vi "STMmyRIO-Server.vi"() -> ()   [LabVIEW 2015]
uses:
  <vilib>/NI/STM/SubVIs/MetaDataElement.ctl
  <vilib>/NI/STM/TCP/TCP Read Options.ctl
  <vilib>/NI/STM/TCP/Write Meta Data (TCP Ref).vi
  <vilib>/NI/STM/TCP/Get Connection Reference (TCP).vi
  <vilib>/NI/STM/TCP/Write Meta Data (TCP Clst).vi
  <vilib>/NI/STM/TCP/Read Message (TCP).vi
  <vilib>/NI/STM/TCP/Write Message (TCP).vi
  <vilib>/NI/STM/NI STM.lvlib
panel:
  out "手动取点y":i32
  out "手动取点x":i32
  out "是否手动取点":bool
  in  "?":bool
  in  "?":bool
  in  "?":bool
  out "触发":bool
  out "自动后退":bool
  out "自动前进":bool
  out "步进距离":u16
  in  "阈值等级":i32=4
  in  "Stop (F)":bool
  in  "关闭程序":bool
  out "error  out":errorcluster
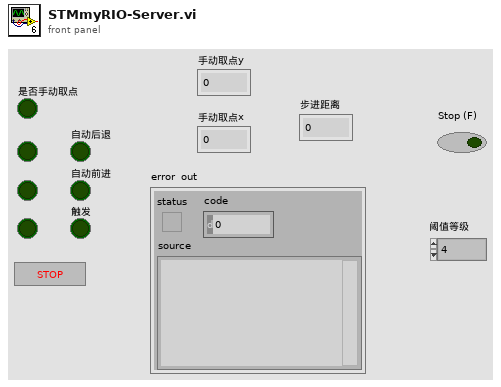
[diagram p1: front panel]
types:
  T1 = typedef "NI STM.lvlib/MetaDataElement.ctl" = string
  T2 = typedef "NI STM.lvlib/TCP Connection Info.ctl" = cluster{"connection ID":refnum<k5>, "meta data":T1[]}
  T3 = cluster{"图像数据":refnum<queue>, "队列输出":refnum<queue>}
  T4 = typedef "IMAQ Image.ctl" = refnum<image>
  T5 = cluster{"滤波":T4, "边缘检测":T4, "untitled":T4, "3D view":T4, "灰度图像":T4}
  T6 = cluster{"周长":dbl, "面积":dbl, "3D":u8[], "灰度图像":T4, "3D view":T4, "滤波":T4, "边缘检测":T4, "3D图像":T4, "质心坐标X":sgl, "质心坐标Y":sgl, "第一点y值，x=0":dbl, "第二点y值，x=639":dbl, "第一点x值，y=0":dbl, "第二点x值，y=479":dbl, "短轴半径um":dbl, "长轴半径um":dbl, "长轴长度":dbl, "短轴长度":dbl, "短轴原曲线":dbl[], "长轴拟合":dbl[], "纵轴拟合":dbl[], "横轴拟合":dbl[], "长轴原曲线":dbl[], "纵轴原曲线":dbl[], "横轴原曲线":dbl[], "短轴拟合":dbl[], "位置":dbl, "触发":bool, "初始化后退":bool, "初始化前进":bool}
  T7 = typedef "NI STM.lvlib/TCP Read Options.ctl" = cluster{"ignore timeout error":bool, "timeout ms (1000)":i32}
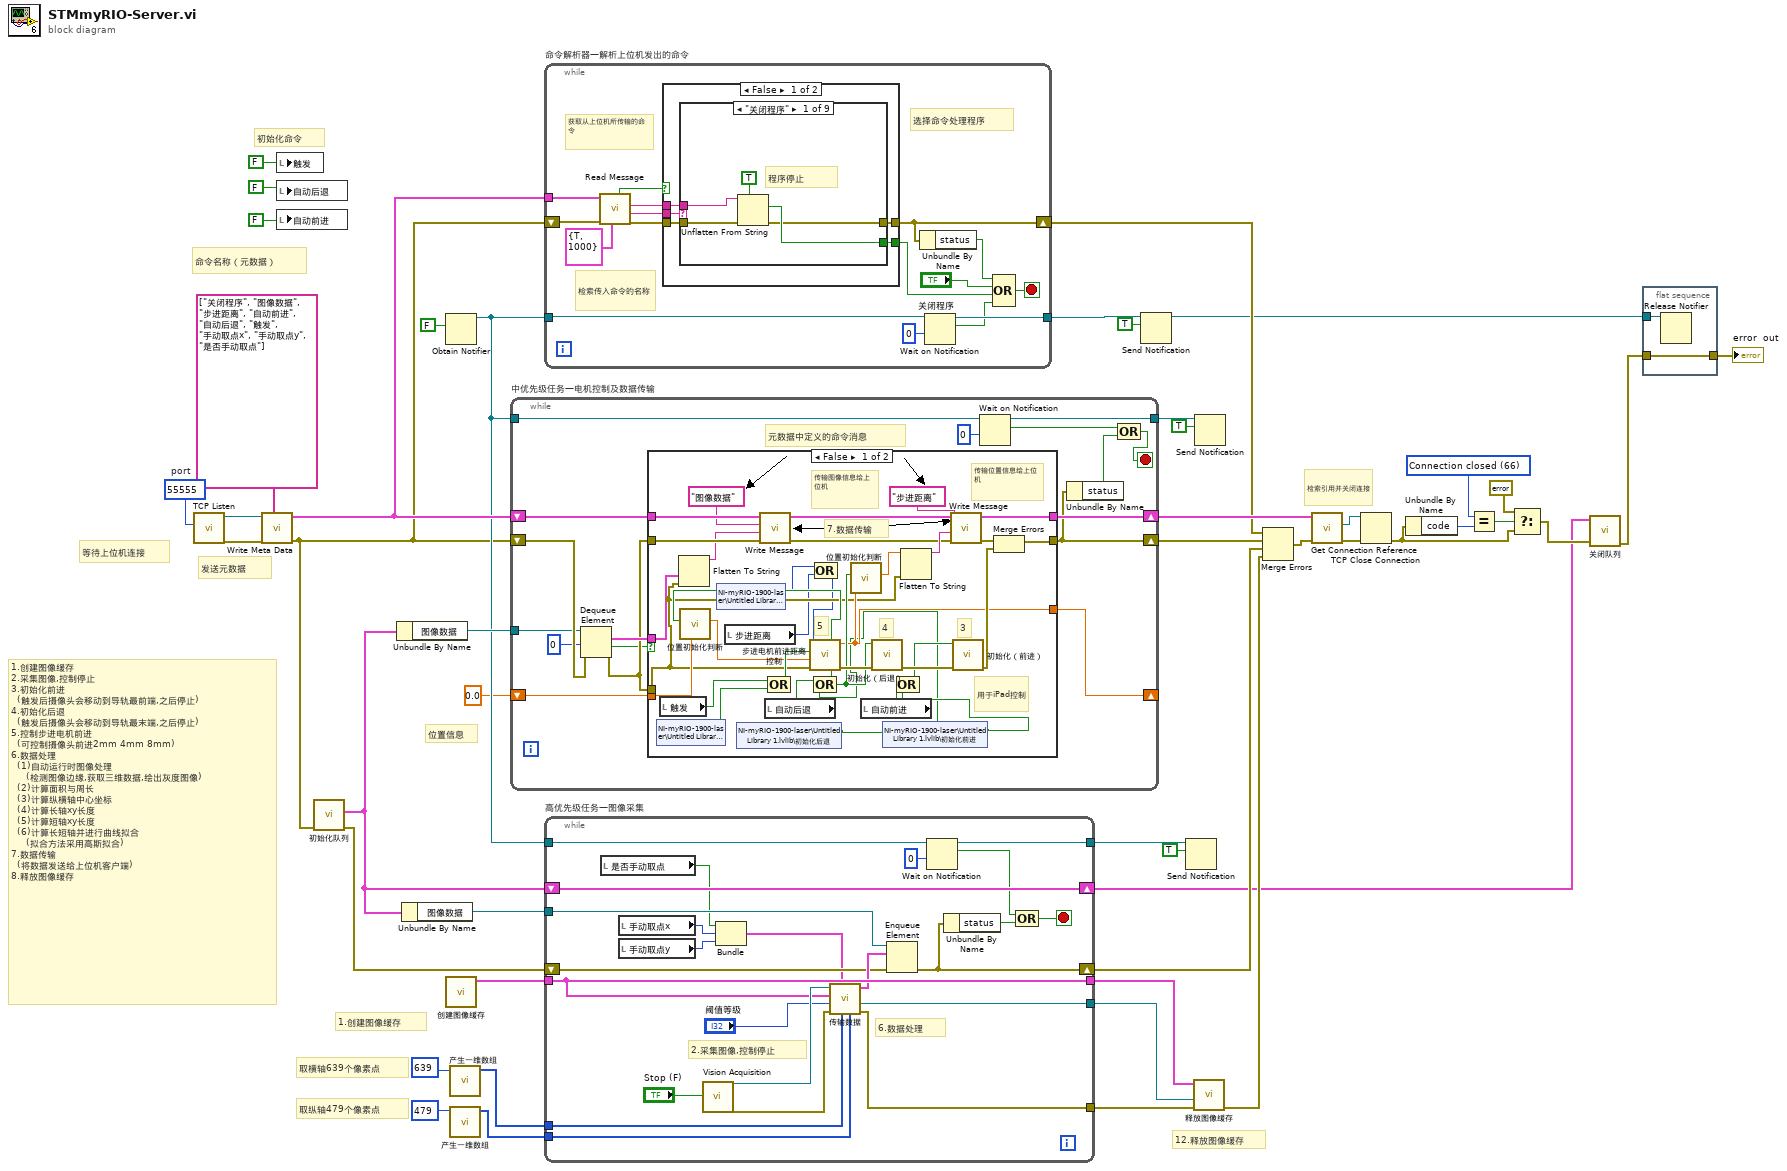
[diagram p0: block diagram]
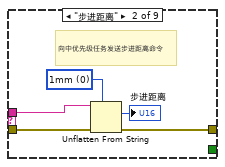
[diagram p3: hidden frame]
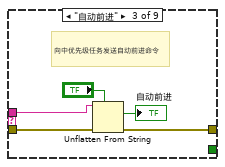
[diagram p4: hidden frame]
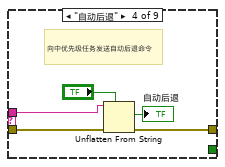
[diagram p5: hidden frame]
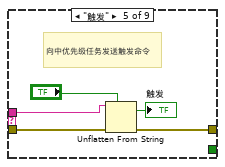
[diagram p6: hidden frame]
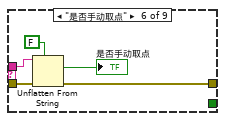
[diagram p7: hidden frame]
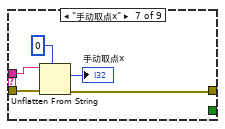
[diagram p8: hidden frame]
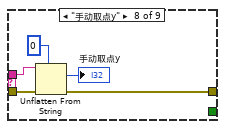
[diagram p9: hidden frame]
diagram:
  w22 = 66 items=["No Error", "Argument Error", "Memory Full", "Out of Zone", "End of File", "File Already Open", "Generic File IO Error", "File Not Found", "File Permission Error", "Disk Full", "Duplicate Path", "Too Many Files Open", "Not Enabled", "Resource File Not Found", "Cannot Add Resource", "Resource Not Found", "Image Not Found", "Image Memory Error", "Pen Does Not Exist", "Config Bad Type", "Config Token Not Found", "Config Parse Error", "Config Memory Error", "Bad External Code Format", "Bad External Code Offset", "External Code Not Present", "Null Window", "Destroy Window Mixup", "Null Menu", "Print Aborted", "Bad Print Record", "Print Driver Error", "Windows Error During Print", "Memory Error During Print", "Print Dialog Error", "Generic Print Error", "Invalid Device Refnum", "Device Not Found", "Device Parameter Error", "Device Unit Error", "Can't Open Device", "Device Call Aborted", "Generic Error", "Cancelled By User", "Object ID Too Low", "Object ID Too High", "Object Not In Heap", "Unknown Heap", "Bad DefProc ID", "DefProc Not In Table", "Message Out Of Range", "Null Method", "Unknown Message", "Manager Call Not Supported", "Bad address", "Connection In progress", "Connection timed out", "Connection is already in progress", "Network attribute not supported", "Network error", "Address in use", "System out of memory", "Connection aborted", "Connection refused", "Connection is not connected", "Connection is already connected", "Connection closed", "Initialize error (interapplication manager)", "Bad occurrence", "Wait on unbound occurrence handler", "Occurrence queue overflow", "Bad path", "Semaphore not signaled", "Unrecognized type (interapplication manager)"] ("1st Error to Convert")
  w48 = u16 55555  # port
  # "位置信息"
  # "初始化命令"
  # "等待上位机连接"
  # "发送元数据"
  # "检索引用并关闭连接"
  # "命令名称（元数据）"
  # "1.创建图像缓存"
  # "1.创建图像缓存\n2.采集图像,控制停止\n3.初始化前进\n  (触发后摄像头会移动到导轨最前端,之后停止)\n4.初始化后退\n  (触发后摄像头会移动到导轨最末端,之后停止)\n5.控制步进电机前进\n  (可控制摄像头前进2mm 4mm 8mm)\n6.数据处理\n  (1)自动运行时图像处理\n     (检测图像边缘,获取三维数据,绘出灰度图像)\n  (2)计算面积与周长\n  (3)计算纵横轴中心坐标\n  (4)计算长轴xy长度\n  (5)计算短轴xy长度\n  (6)计算长短轴并进行曲线拟合\n     (拟合方法采用高斯拟合) \n7.数据传输 \n  (将数据发送给上位机客户端) \n8.释放图像缓存"
  # "取纵轴479个像素点"
  # "取横轴639个像素点"
  # "12.释放图像缓存"
  n1 = call <vilib>:"TCP Listen.vi"("port"=w48) -> ("error out"=w46:errorcluster, "connection ID"=w47:refnum<k5>)  [unwired: 3 in, 6 out]
  n2 = call-poly "Write Meta Data.vi"("meta data"=T1[] ["关闭程序", "图像数据", "步进距离", "自动前进", "自动后退", "触发", "手动取点x", "手动取点y", "是否手动取点"] ("Meta data"), "error in"=w46, "connection ID"=w47) -> ("error out"=w19:errorcluster, "connection info out"=w45:T2)  [unwired: 2 in, 5 out]
  n3 = local write "触发"(FALSE) -> ()
  n4 = local write "自动后退"(FALSE) -> ()
  n5 = local write "自动前进"(FALSE) -> ()
  n6 = call "初始化队列.vi"("error in (no error)"=w19) -> ("error out"=w18:errorcluster, "输出簇"=w1:T3)  [unwired: 9 in]
  n7 = Unbundle By Name(w1) -> ("图像数据"=w44:refnum<queue>)
  n8 = Unbundle By Name(w1) -> ("图像数据"=w43:refnum<queue>)
  n9 = Obtain Notifier(notification data type=FALSE) -> (notifier out=w29:refnum<notifier>)  [unwired: 3 in, 2 out]
  n10 = call "创建图像缓存.vi"() -> ("簇"=w17:T5)  [unwired: 11 in]
  n11 = call "产生一维数组.vi"("Numeric"=639) -> ("Array"=w8:i32[])  [unwired: 10 in]
  n12 = call "产生一维数组.vi"("Numeric"=479) -> ("Array"=w7:i32[])  [unwired: 10 in]
  n13 = while "中优先级任务—电机控制及数据传输" {
    tunnel: w44 -> [w56]
    shift-right: [w58] -> w39
    shift-left: w19 -> [w62]
    shift-right: [w64] -> w42
    shift-left: w45 -> [w65]
    tunnel: w29 -> [w59]
    tunnel: [w57] -> w30
    shift-right: [w54] -> _
    shift-left: 0.0 ("x") -> [w55]
    stop <- w49 stop-if-true
    # "元数据中定义的命令消息"
    n14 = Dequeue Element(queue=w56, timeout in ms (-1)=0, error in (no error)=w62) -> (element=w63:T6, timed out?=w52:bool, error out=w53:errorcluster)  [unwired: 1 out]
    n15 = case shown="False" w52 {
      tunnel: w65 -> [w97 w100]
      tunnel: w53 -> [w96 w99]
      tunnel: [w89 w100] -> w64
      tunnel: [w84 w99] -> w58
      tunnel: w63 -> [w83 _]
      tunnel: w55 -> [w76 w98]
      tunnel: [w73 w98] -> w54
      tunnel: w53 -> [w71 _]
      frame False {
        # "传输图像信息给上位机"
        # "用于iPad控制"
        # "传输位置信息给上位机"
        # "7.数据传输"
        # "3"
        # "4"
        # "5"
        n16 = shared-variable "NI-myRIO-1900-laser\\Untitled Library 1.lvlib\\触发"() -> (w81:bool)  [unwired: 1 in, 1 out]
        n17 = local read "触发"() -> (w82:bool)
        n18 = Flatten To String(anything=w83, error in (no error)=w71) -> (data string=w94:string)  [unwired: 4 out]
        n19 = shared-variable "NI-myRIO-1900-laser\\Untitled Library 1.lvlib\\枚举"() -> (w66:i8)  [unwired: 1 in, 1 out]
        n20 = local read "步进距离"() -> (w68:u16)
        n21 = shared-variable "NI-myRIO-1900-laser\\Untitled Library 1.lvlib\\初始化后退"() -> (w69:bool)  [unwired: 1 in, 1 out]
        n22 = call-poly "Write Message.vi"("error in"=w96, "data"=w94, "name"="图像数据" ("Name"), "connection info in"=w97) -> ("error out"=w90:errorcluster, "connection info out"=w91:T2)  [unwired: 1 in, 5 out]
        n23 = local read "自动后退"() -> (w79:bool)
        n24 = Compound Arithmetic op=OR(w82, w81) -> (w80:bool)
        n25 = Compound Arithmetic op=OR(w79, w69) -> (w74:bool)
        n26 = call "位置初始化判断.vi"("位置初始化"=w76, "是否后退"=w74) -> ("位置判断"=w75:dbl)  [unwired: 9 in]
        n27 = Compound Arithmetic op=OR(w66, w68) -> (w67:u16)
        n28 = call "步进电机前进距离控制.vi"("error in"=w71, "初始化位置"=w75, "触发"=w80, "枚举"=w67) -> ("error out"=w88:errorcluster, "位置"=w73:dbl)  [unwired: 6 in]
        n29 = call "位置初始化判断.vi"("位置初始化"=w73, "是否后退"=w74) -> ("位置判断"=w72:dbl)  [unwired: 9 in]
        n30 = local read "自动前进"() -> (w78:bool)
        n31 = call "初始化（后退）.vi"("error in"=w88, "初始化"=w74) -> ("error out"=w87:errorcluster)  [unwired: 9 in]
        n32 = shared-variable "NI-myRIO-1900-laser\\Untitled Library 1.lvlib\\初始化前进"() -> (w70:bool)  [unwired: 1 in, 1 out]
        n33 = Compound Arithmetic op=OR(w78, w70) -> (w77:bool)
        n34 = Flatten To String(anything=w72, error in (no error)=w71) -> (data string=w93:string)  [unwired: 4 out]
        n35 = call-poly "Write Message.vi"("error in"=w90, "data"=w93, "name"="步进距离" ("Name"), "connection info in"=w91) -> ("error out"=w86:errorcluster, "connection info out"=w89:T2)  [unwired: 1 in, 5 out]
        n36 = call "初始化（前进）.vi"("error in"=w87, "初始化"=w77) -> ("error out"=w85:errorcluster)  [unwired: 9 in]
        n37 = Merge Errors(w86, w85) -> (w84:errorcluster)
      }
      frame True {
      }
    }
    n38 = Wait on Notification(notifier=w59, timeout in ms (-1)=0) -> (notifier out=w57:refnum<notifier>, notification=w51:bool)  [unwired: 2 in, 2 out]
    n39 = Unbundle By Name(w58) -> ("status"=w50:bool)
    n40 = Compound Arithmetic op=OR(w51, w50) -> (w49:bool)
  }
  n41 = while "命令解析器—解析上位机发出的命令" {
    tunnel: w45 -> [w116]
    shift-right: [w107] -> w37
    shift-left: w19 -> [w115]
    tunnel: w29 -> [w109]
    tunnel: [w103] -> w33
    stop <- w104 stop-if-true
    # "选择命令处理程序"
    # "检索传入命令的名称"
    # "获取从上位机所传输的命令"
    n42 = call-poly <vilib>:"Read Message.vi"("options"=T7 {"ignore timeout error"=TRUE, "timeout ms (1000)"=1000} ("Options"), "error in"=w115, "connection info in"=w116) -> ("error out"=w111:errorcluster, "name"=w114:T1, "data string"=w113:string, "timed out?"=w112:bool)  [unwired: 2 in, 3 out]
    n43 = case shown="False" w112 {
      tunnel: w114 -> [w117 _]
      tunnel: w113 -> [w121 _]
      tunnel: w111 -> [w120 w163]
      tunnel: [w119 w163] -> w107
      tunnel: [w118 _] -> w101
      frame False {
        n44 = case shown="\"关闭程序\"" w117 {
          tunnel: w121 -> [w125 w128 w135 w140 w145 w150 w154 w161 _]
          tunnel: w120 -> [w124 w131 w136 w141 w146 w149 w155 w160 w162]
          tunnel: [w122 w130 w134 w139 w144 w147 w153 w158 w162] -> w119
          tunnel: [w123 _ _ _ _ _ _ _ _] -> w118
          frame "关闭程序" {
            # "程序停止"
            n45 = Unflatten From String(type=TRUE, binary string=w125, error in (no error)=w124) -> (value=w123:bool, error out=w122:errorcluster)  [unwired: 1 in, 2 out]
          }
          frame "步进距离" {
            w129 = u16 0 items=["1mm", "2mm", "4mm", "8mm"] ("步进距离")
            # "向中优先级任务发送步进距离命令"
            n46 = Unflatten From String(type=w129, binary string=w128, error in (no error)=w131) -> (value=→"步进距离":u16, error out=w130:errorcluster)  [unwired: 1 in, 2 out]
          }
          frame "自动前进" {
            # "向中优先级任务发送自动前进命令"
            n47 = Unflatten From String(type="?", binary string=w135, error in (no error)=w136) -> (value=→"自动前进":bool, error out=w134:errorcluster)  [unwired: 1 in, 2 out]
          }
          frame "自动后退" {
            # "向中优先级任务发送自动后退命令"
            n48 = Unflatten From String(type="?", binary string=w140, error in (no error)=w141) -> (value=→"自动后退":bool, error out=w139:errorcluster)  [unwired: 1 in, 2 out]
          }
          frame "触发" {
            # "向中优先级任务发送触发命令"
            n49 = Unflatten From String(type="?", binary string=w145, error in (no error)=w146) -> (value=→"触发":bool, error out=w144:errorcluster)  [unwired: 1 in, 2 out]
          }
          frame "是否手动取点" {
            n50 = Unflatten From String(type=FALSE, binary string=w150, error in (no error)=w149) -> (value=→"是否手动取点":bool, error out=w147:errorcluster)  [unwired: 1 in, 2 out]
          }
          frame "手动取点x" {
            n51 = Unflatten From String(type=0 ("新值"), binary string=w154, error in (no error)=w155) -> (value=→"手动取点x":i32, error out=w153:errorcluster)  [unwired: 1 in, 2 out]
          }
          frame "手动取点y" {
            n52 = Unflatten From String(type=0 ("新值"), binary string=w161, error in (no error)=w160) -> (value=→"手动取点y":i32, error out=w158:errorcluster)  [unwired: 1 in, 2 out]
          }
          frame Default {
          }
        }
      }
      frame True {
      }
    }
    n53 = Unbundle By Name(w107) -> ("status"=w106:bool)
    n54 = Wait on Notification(notifier=w109, timeout in ms (-1)=0) -> (notifier out=w103:refnum<notifier>, notification=w102:bool)  [unwired: 2 in, 2 out]
    n55 = Compound Arithmetic op=OR(w106, "关闭程序", w101, w102) -> (w104:bool)
  }
  n56 = while "高优先级任务—图像采集" {
    tunnel: w43 -> [w187]
    shift-right: [w183] -> w38
    shift-left: w18 -> [w168]
    shift-right: [w186] -> w5
    shift-left: w1 -> [w186]
    tunnel: w29 -> [w184]
    tunnel: [w179] -> w27
    tunnel: [w174] -> w16
    tunnel: [w173] -> w15
    tunnel: w8 -> [w171]
    tunnel: w7 -> [w170]
    tunnel: w17 -> [w172]
    tunnel: [w172] -> w14
    stop <- w180 stop-if-true
    # "6.数据处理"
    # "2.采集图像,控制停止"
    n57 = local read "是否手动取点"() -> (w167:bool)
    n58 = local read "手动取点x"() -> (w166:i32)
    n59 = local read "手动取点y"() -> (w165:i32)
    n60 = call "Vision Acquisition"("Stop (F)"="Stop (F)") -> ("Image Out"=w178:T4, "error out"=w177:errorcluster)  [unwired: 22 in, 3 out]
    n61 = Bundle("是否手动取点"=w167, "手动取点x"=w166, "手动取点y"=w165) -> (w164:cluster{"是否手动取点":bool, "手动取点x":i32, "手动取点y":i32})  [unwired: 1 in]
    n62 = call "传输数据.vi"("纵轴数组"=w170, "横纵数组"=w171, "输出簇"=w164, "error in (no error)"=w177, "阈值等级"="阈值等级", "配置缓存"=w172, "Image Src"=w178) -> ("error out"=w174:errorcluster, "灰度图像"=w173:T4, "已采集数据"=w169:T6)  [unwired: 2 in]
    n63 = Enqueue Element(queue=w187, element=w169, error in (no error)=w168) -> (error out=w183:errorcluster)  [unwired: 3 out]
    n64 = Wait on Notification(notifier=w184, timeout in ms (-1)=0) -> (notifier out=w179:refnum<notifier>, notification=w181:bool)  [unwired: 2 in, 2 out]
    n65 = Unbundle By Name(w183) -> ("status"=w182:bool)
    n66 = Compound Arithmetic op=OR(w181, w182) -> (w180:bool)
  }
  n67 = Send Notification(notification=TRUE, notifier=w33) -> (notifier out=w26:refnum<notifier>)  [unwired: 1 in, 1 out]
  n68 = Send Notification(notification=TRUE, notifier=w27) -> ()  [unwired: 1 in, 2 out]
  n69 = call "释放图像缓存.vi"("错误输入（无错误）"=w16, "灰度图像"=w15, "缓存数据"=w14) -> ("错误输出"=w13:errorcluster)  [unwired: 8 in]
  n70 = Send Notification(notification=TRUE, notifier=w30) -> ()  [unwired: 1 in, 2 out]
  n71 = Merge Errors(w37, w39, w38, w13) -> (w36:errorcluster)
  n72 = call-poly <vilib>:"Get Connection Reference.vi"("error in"=w36, "connection info in"=w42) -> ("error out"=w40:errorcluster, "connection ID out"=w41:refnum<k5>)  [unwired: 8 out]
  n73 = TCP Close Connection(connection ID=w41, error in (no error)=w40) -> (error out=w21:errorcluster)  [unwired: 2 out]
  n74 = Unbundle By Name(w21) -> ("code"=w24:i32)
  n75 = Equal?(x=w22, y=w24) -> (x = y?=w23:bool)
  n76 = Select(t=errorcluster {"status"=FALSE, "code"=0, "source"=""}, s=w23, f=w21) -> (s? t:f=w12:errorcluster)
  n77 = call "关闭队列.vi"("error in (no error)"=w12, "输出簇"=w5) -> ("error out"=w11:errorcluster)  [unwired: 9 in]
  n78 = flat-sequence {
    tunnel: w26 -> [w189]
    tunnel: w11 -> [w188]
    tunnel: [w188] -> w25
    frame #0 {
      n79 = Release Notifier(notifier=w189) -> ()  [unwired: 2 in, 3 out]
    }
  }
  "error  out" <- w25
